vi "prova resistomat.vi"() -> ()   [LabVIEW 2016]
panel:
  out "error out":errorcluster {"code" format="%.0x"}
  out "Instrument ID":i32
  in  "COM-Port (0)":i32=2 min=1 max=32 step=1
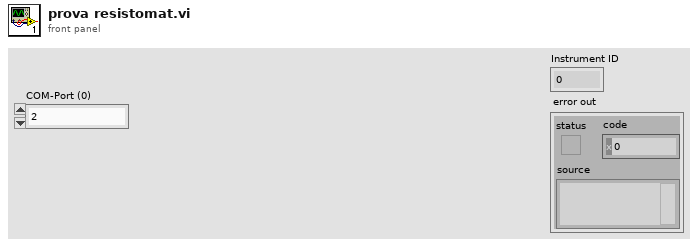
[diagram p1: front panel]
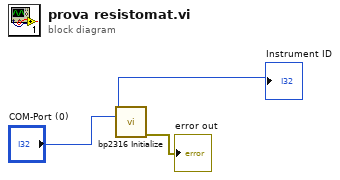
[diagram p0: block diagram]
diagram:
  n1 = call <instrlib>:"bp2316 Initialize.vi"("COM-Port (0)"="COM-Port (0)") -> ("Instrument ID"=→"Instrument ID":i32, "error out"=→"error out":errorcluster)  [unwired: 12 in, 1 out]
